vi "INA219 Config2Code.vi"(11 "INA219 Config Options":T1={"I2C"={"Slave Address"=64, "Channel"=0}, "Reset bit"=0, "Bus Voltage Range"=1, "PGA/Shunt Voltage Gain"=3, "Bus Voltage ADC Settings"=8, "Shunt Voltage ADC Settings"=3, "Mode"=7, "Calibration Value"=4096, "Online"=FALSE} {"I2C"."Slave Address" format="%.0x"; "Calibration Value" format="%.0x"; "Mode" items=["Power Down", "Shunt Voltage, Triggered", "Bus Voltage, Triggered", "Shunt & Bus, Triggered", "ADC Off (Disabled)", "Shunt Voltage, Continuous", "Bus Voltage, Continuous", "Shunt & Bus Voltage, Continuous"]; "Shunt Voltage ADC Settings" items=["9-bit, 84us conversion time"=0, "10-bit, 148us conversion time"=1, "11-bit, 276us conversion time"=2, "12-bit, 532us conversion time"=3, "1x12-bit, 532us conversion time"=8, "2x12-bit averaged, 1.06ms conversion time"=9, "4x12-bit averaged, 2.13ms conversion time"=10, "8x12-bit averaged, 4.26ms conversion time"=11, "16x12-bit averaged, 8.51ms conversion time"=12, "32x12-bit averaged, 17.02ms conversion time"=13, "64x12-bit averaged, 34.05ms conversion time"=14, "128x12-bit averaged, 68.10ms conversion time"=15]; "Bus Voltage ADC Settings" items=["9-bit, 84us conversion time"=0, "10-bit, 148us conversion time"=1, "11-bit, 276us conversion time"=2, "12-bit, 532us conversion time"=3, "1x12-bit, 532us conversion time"=8, "2x12-bit averaged, 1.06ms conversion time"=9, "4x12-bit averaged, 2.13ms conversion time"=10, "8x12-bit averaged, 4.26ms conversion time"=11, "16x12-bit averaged, 8.51ms conversion time"=12, "32x12-bit averaged, 17.02ms conversion time"=13, "64x12-bit averaged, 34.05ms conversion time"=14, "128x12-bit averaged, 68.10ms conversion time"=15]; "PGA/Shunt Voltage Gain" items=["Gain 1, +/-40mV", "Gain 2, +/-80mV", "Gain 3, +/-160mV", "Gain 4, +/-320mV"]; "Bus Voltage Range" items=["0-16V Range", "0-32V Range"]; "Reset bit" items=["Do Not Reset", "Reset"]}) -> (3 "Config Code":u16 format="%04x")   [LabVIEW 2014]
uses:
  INA219 Config Options.ctl
panel:
  out "Config (binary)":bool[](array[boolean])
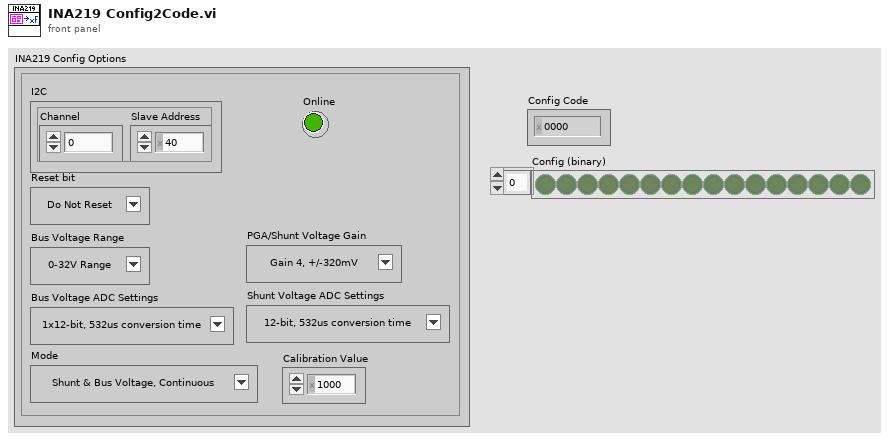
[diagram p1: front panel]
types:
  T1 = typedef "INA219 Config Options.ctl" = cluster{"I2C":cluster{"Slave Address":u8, "Channel":u8}, "Reset bit":u8, "Bus Voltage Range":u8, "PGA/Shunt Voltage Gain":u8, "Bus Voltage ADC Settings":u8, "Shunt Voltage ADC Settings":u8, "Mode":u8, "Calibration Value":u16, "Online":bool}
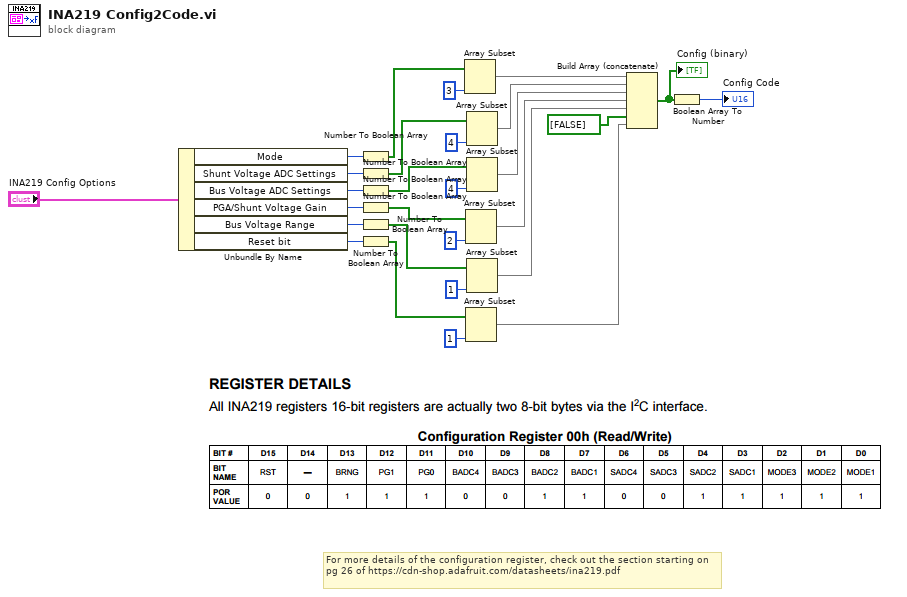
[diagram p0: block diagram]
diagram:
  # "For more details of the configuration register, check out the section starting on pg 26 of https://cdn-shop.adafruit.com/datasheets/ina219.pdf"
  n1 = Unbundle By Name("INA219 Config Options") -> ("Mode"=w27:u8, "Shunt Voltage ADC Settings"=w22:u8, "Bus Voltage ADC Settings"=w26:u8, "PGA/Shunt Voltage Gain"=w25:u8, "Bus Voltage Range"=w24:u8, "Reset bit"=w23:u8)
  n2 = Number To Boolean Array(number=w27) -> (Boolean array=w13:bool[])
  n3 = Number To Boolean Array(number=w22) -> (Boolean array=w12:bool[])
  n4 = Number To Boolean Array(number=w26) -> (Boolean array=w11:bool[])
  n5 = Number To Boolean Array(number=w25) -> (Boolean array=w10:bool[])
  n6 = Number To Boolean Array(number=w24) -> (Boolean array=w9:bool[])
  n7 = Number To Boolean Array(number=w23) -> (Boolean array=w8:bool[])
  n8 = Array Subset(array=w13, length=3) -> (w3:bool[])  [unwired: 1 in]
  n9 = Array Subset(array=w10, length=2) -> (w6:bool[])  [unwired: 1 in]
  n10 = Array Subset(array=w8, length=1) -> (w2:bool[])  [unwired: 1 in]
  n11 = Array Subset(array=w12, length=4) -> (w4:bool[])  [unwired: 1 in]
  n12 = Array Subset(array=w11, length=4) -> (w5:bool[])  [unwired: 1 in]
  n13 = Array Subset(array=w9, length=1) -> (w7:bool[])  [unwired: 1 in]
  n14 = Build Array (concatenate)(w3, w4, w5, w6, w7, bool[] [FALSE] ("element"), w2) -> (w15:bool[])
  "Config (binary)" <- w15
  n15 = Boolean Array To Number(Boolean array=w15) -> (number=→"Config Code":u16)
